vi "decode point message.vi"(11 "input stream":u8) -> (0 "y value":i16, 1 "x value":i16, 2 "new y":bool=TRUE, 3 "new x":bool=TRUE, 4 "waiting for new message":bool)   [LabVIEW 2009]
uses:
  vision decoder state typedef.ctl
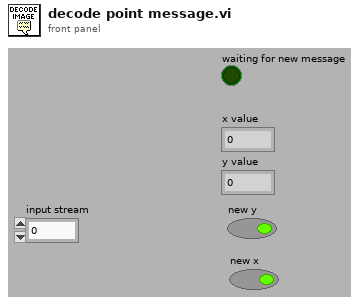
[diagram p1: front panel]
types:
  T1 = typedef "vision decoder state typedef.ctl" = enum16{"wait for message start '['", "wait for point start '(' ", "record x value", "record y value", "scan complete"}
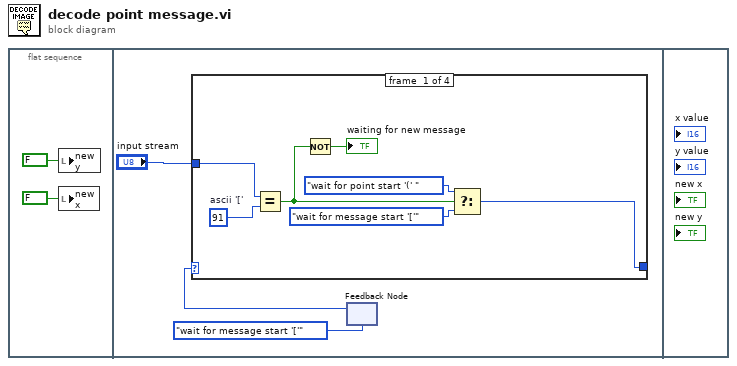
[diagram p0: block diagram]
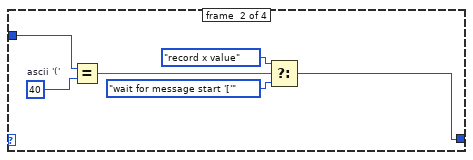
[diagram p2: hidden frame]
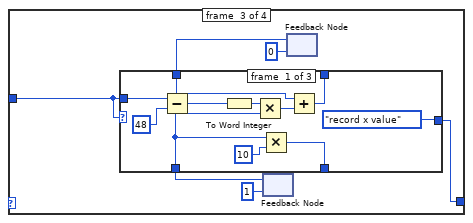
[diagram p3: hidden frame]
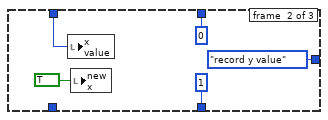
[diagram p4: hidden frame]
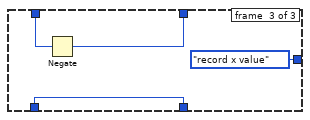
[diagram p5: hidden frame]
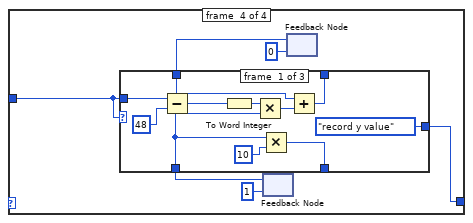
[diagram p6: hidden frame]
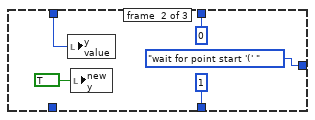
[diagram p7: hidden frame]
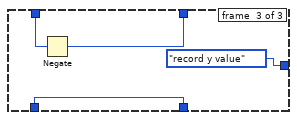
[diagram p8: hidden frame]
diagram:
  n1 = flat-sequence {
    frame #0 {
      n2 = local write "new y"(FALSE) -> ()
      n3 = local write "new x"(FALSE) -> ()
    }
    frame #1 {
      n4 = feedback #1(vision_decoder_state_typedef."wait for message start '['" ("Enum")) -> (w5:T1)
      n5 = case shown="\"wait for message start '['\", Default" w5 {
        tunnel: "input stream" -> [w12 w18 w21 w49]
        tunnel: [w8 w14 w20 w48] -> w3
        frame #0 {
          w13 = u8 91  # ascii '['
          n6 = Equal?(x=w12, y=w13) -> (x = y?=w11:bool)
          n7 = Not(x=w11) -> (.not. x?=→"waiting for new message":bool)
          n8 = Select(t=vision_decoder_state_typedef."wait for point start '(' " ("Enum"), s=w11, f=vision_decoder_state_typedef."wait for message start '['" ("Enum")) -> (s? t:f=w8:T1)
        }
        frame #1 {
          w19 = u8 40  # ascii '('
          n9 = Equal?(x=w18, y=w19) -> (x = y?=w17:bool)
          n10 = Select(t=vision_decoder_state_typedef."record x value" ("Enum"), s=w17, f=vision_decoder_state_typedef."wait for message start '['" ("Enum")) -> (s? t:f=w14:T1)
        }
        frame #2 {
          n11 = feedback #2(i16 1) -> (w25:i16)
          n12 = feedback #3(i16 0) -> (w22:i16)
          n13 = case shown="45" w21 {
            tunnel: w21 -> [w38 _ _]
            tunnel: [w34 i16 1 w44] -> w27
            tunnel: w25 -> [w33 _ w44]
            tunnel: [w30 i16 0 w45] -> w24
            tunnel: w22 -> [w29 w41 w47]
            tunnel: [vision_decoder_state_typedef."record x value" ("Enum") vision_decoder_state_typedef."record y value" ("Enum") vision_decoder_state_typedef."record x value" ("Enum")] -> w20
            frame #0 {
              n14 = Subtract(x=w38, y=u8 48) -> (x-y=w36:u8)
              n15 = To Word Integer(number=w36) -> (16bit integer=w32:i16)
              n16 = Multiply(x=w32, y=w33) -> (x*y=w31:i16)
              n17 = Multiply(x=w33, y=i16 10) -> (x*y=w34:i16)
              n18 = Add(x=w29, y=w31) -> (x+y=w30:i16)
            }
            frame #1 {
              n19 = local write "x value"(w41) -> ()
              n20 = local write "new x"(TRUE) -> ()
            }
            frame #2 {
              n21 = Negate(x=w47) -> (-x=w45:i16)
            }
          }
        }
        frame #3 {
          n22 = feedback #4(i16 1) -> (w53:i16)
          n23 = feedback #5(i16 0) -> (w50:i16)
          n24 = case shown="45" w49 {
            tunnel: w49 -> [w66 _ _]
            tunnel: [w62 i16 1 w72] -> w55
            tunnel: w53 -> [w61 _ w72]
            tunnel: [w58 i16 0 w73] -> w52
            tunnel: w50 -> [w57 w69 w75]
            tunnel: [vision_decoder_state_typedef."record y value" ("Enum") vision_decoder_state_typedef."wait for point start '(' " ("Enum") vision_decoder_state_typedef."record y value" ("Enum")] -> w48
            frame #0 {
              n25 = Subtract(x=w66, y=u8 48) -> (x-y=w64:u8)
              n26 = To Word Integer(number=w64) -> (16bit integer=w60:i16)
              n27 = Multiply(x=w60, y=w61) -> (x*y=w59:i16)
              n28 = Multiply(x=w61, y=i16 10) -> (x*y=w62:i16)
              n29 = Add(x=w57, y=w59) -> (x+y=w58:i16)
            }
            frame #1 {
              n30 = local write "y value"(w69) -> ()
              n31 = local write "new y"(TRUE) -> ()
            }
            frame #2 {
              n32 = Negate(x=w75) -> (-x=w73:i16)
            }
          }
        }
      }
    }
    frame #2 {
    }
  }
